vi "Write Key.vi"   [LabVIEW 2024, in "Generic Config Handling.lvlib"]
doc: "This vi writes a variant to a config file.\n\nIt only accepts very basic datatypes. \n\nIt will accept 1D and 2D arrays.\n\nIf key name is not wired, then it will use the name of the section element."
uses:
  Generic Config Handling.lvlib
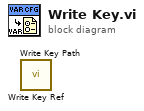
[diagram p0: block diagram]
diagram:
  n1 = call "Write Key Ref.vi"() -> ()  [unwired: 10 in, 2 out]
  n2 = call "Write Key Path.vi"() -> ()  [unwired: 9 in, 3 out]
